vi "get support folder path.vi"() -> (0 "support folder path":path)   [LabVIEW 2020, in "main.lvlib"]
uses:
  main.lvlib
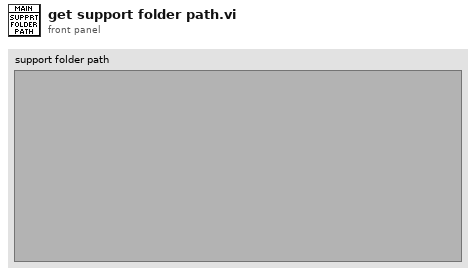
[diagram p1: front panel]
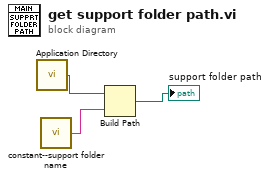
[diagram p0: block diagram]
diagram:
  n1 = call <vilib>:"Application Directory.vi"() -> ("Application Directory"=w3:path)
  n2 = call "constant--support folder name.vi"() -> ("Name of support folder"=w2:string)
  n3 = Build Path(base path=w3, name or relative path=w2) -> (appended path=→"support folder path":path)
